vi "Test-Number Count Down.vi"() -> ()   [LabVIEW 2017]
uses:
  user.lib/NEVSTOP-Programming-Palette/Signal/_Instance/_Number Count Down(Array).vi
  user.lib/NEVSTOP-Programming-Palette/Signal/_Instance/_Number Count Down(Element).vi
  user.lib/NEVSTOP-Programming-Palette/Signal/_Instance/_Number Count Down(Array).vi/9de0e42d-c65c-4cbc-a92d-661ac054e2ac.vi
panel:
  in  "Valid?(T)":bool=TRUE
  in  "Numeric 3":i32[](array[numeric])=[16, 15]
  in  "Numeric 2":i32=15
  in  "Numeric 1":i32=16
  in  "threasholds":i64=1000
  out "left 3":i64[](array[numeric])
  out "left 1":i64
  out "left 2":i64
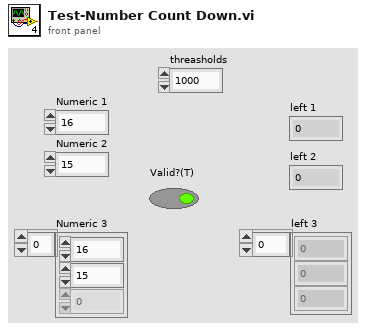
[diagram p1: front panel]
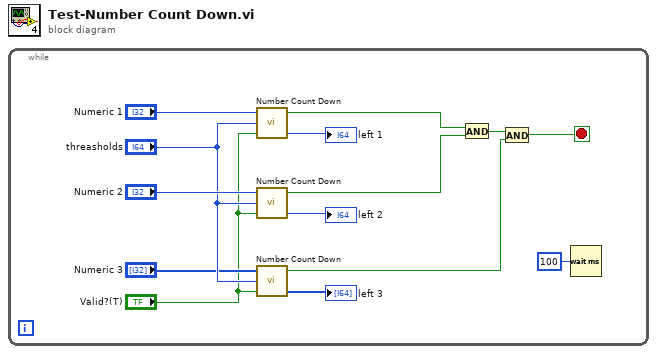
[diagram p0: block diagram]
diagram:
  n1 = while {
    stop <- w4 stop-if-true
    n2 = call-poly "Number Count Down.vi"("number"="Numeric 1", "threashold"="threasholds", "Valid?(T)"="Valid?(T)") -> ("reach?"=w12:bool, "left"=→"left 1":i64)  [unwired: 5 in]
    n3 = call-poly "Number Count Down.vi"("number"="Numeric 2", "threashold"="threasholds", "Valid?(T)"="Valid?(T)") -> ("reach?"=w11:bool, "left"=→"left 2":i64)  [unwired: 5 in]
    n4 = call-poly "Number Count Down.vi"("fixed size array"="Numeric 3", "threashold"="threasholds", "Valid?(T)"="Valid?(T)") -> ("reach?"=w2:bool, "left"=→"left 3":i64[])  [unwired: 5 in]
    n5 = And(x=w12, y=w11) -> (x .and. y?=w3:bool)
    n6 = And(x=w3, y=w2) -> (x .and. y?=w4:bool)
    n7 = Wait (ms)(milliseconds to wait=u32 100) -> ()  [unwired: 1 out]
  }
